vi "Begin BidirectionalStreamTemplate.vi"(8 "error in":errorcluster, 9 "timeoutMs":i32=-1, 11 "gRPC ID":T1) -> (0 "error out":errorcluster, 2 "Call Id Out":T1, 3 "gRPC ID out":T1)   [LabVIEW 2019, in "Client Template.lvlib"]
uses:
  Client Template.lvlib
  <vilib>/gRPC/LabVIEW gRPC Library/Shared/grpcId.ctl
  <vilib>/gRPC/LabVIEW gRPC Library/gprc-lvsupport-release.lvlib
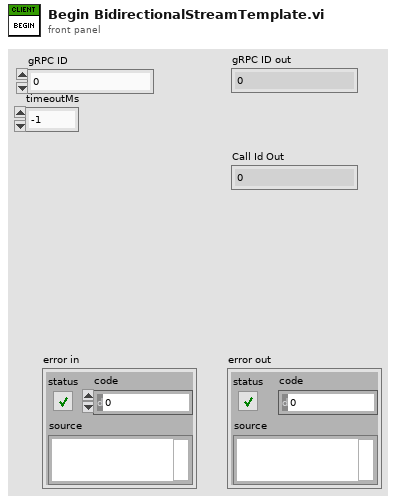
[diagram p1: front panel]
types:
  T1 = typedef "gprc-lvsupport-release.lvlib/grpcId.ctl" = u64
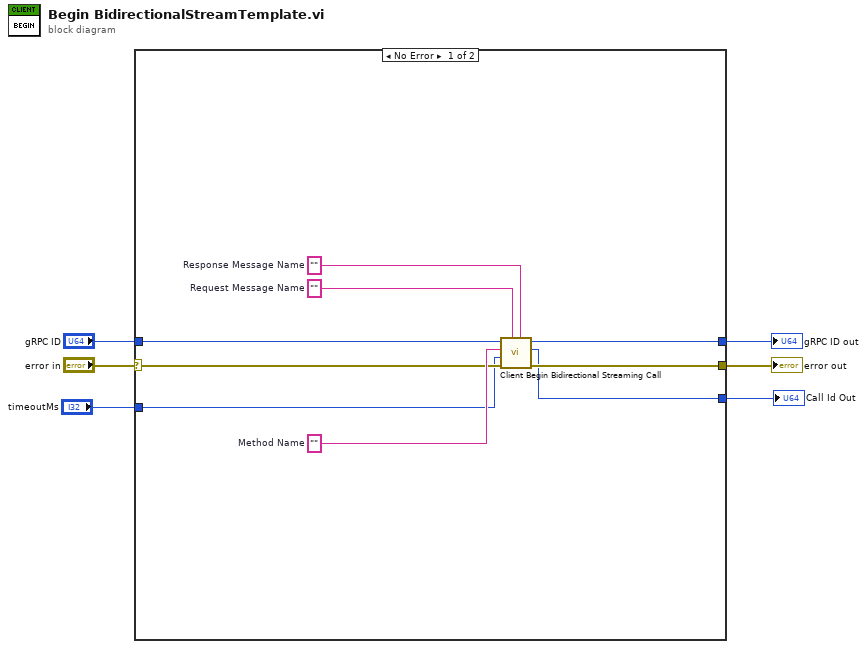
[diagram p0: block diagram]
diagram:
  n1 = case shown="No Error" "error in" {
    selector: "error in" -> [w12 w16]
    tunnel: [w11 w16] -> w5
    tunnel: "gRPC ID" -> [w10 w17]
    tunnel: [w9 w17] -> w3
    tunnel: [w8 _] -> w2
    tunnel: "timeoutMs" -> [w7 _]
    frame No Error {
      w13 = ""  # Response Message Name
      w14 = ""  # Request Message Name
      w15 = ""  # Method Name
      n2 = call <vilib>:"Client Begin Bidirectional Streaming Call.vi"("Response Message Name"=w13, "Request Message Name"=w14, "error in"=w12, "timeoutMs"=w7, "Method Name"=w15, "ClientID in"=w10) -> ("error out"=w11:errorcluster, "Call ID out"=w8:T1, "ClientID out"=w9:T1)  [unwired: 3 in]
    }
    frame Error {
    }
  }
  "error out" <- w5
  "gRPC ID out" <- w3
  "Call Id Out" <- w2
